vi "GetInfoForVIParser.vi"(5 "Data Types":string[](array[string]), 6 "OutputIdx":i32[](array[numeric]), 7 "InputIdx":i32[](array[numeric]), 8 "Dirs":T1[](array[typedef]), 9 "Param Names":string[](array[string])) -> (0 "OutputIdx Out":i32[](array[numeric]), 1 "InputIdx Out":i32[](array[numeric]), 2 "Dirs Out":T1[](array[typedef]), 3 "ParamNames Out":string[](array[string]), 4 "DataTypesOut":string[](array[string]))   [LabVIEW 2020]
uses:
  <vilib>/AppBuilder/IOStatus.ctl
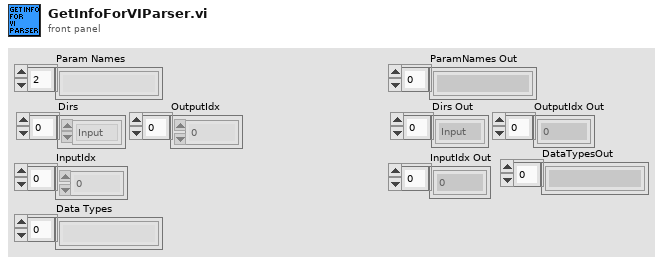
[diagram p1: front panel]
types:
  T1 = typedef "IOStatus.ctl" = enum16{"Input", "Output", "Input/Output", "InputDeleted", "OutputDeleted", "IODeleted", "ErrorClusterIn", "ErrorClusterOut"}
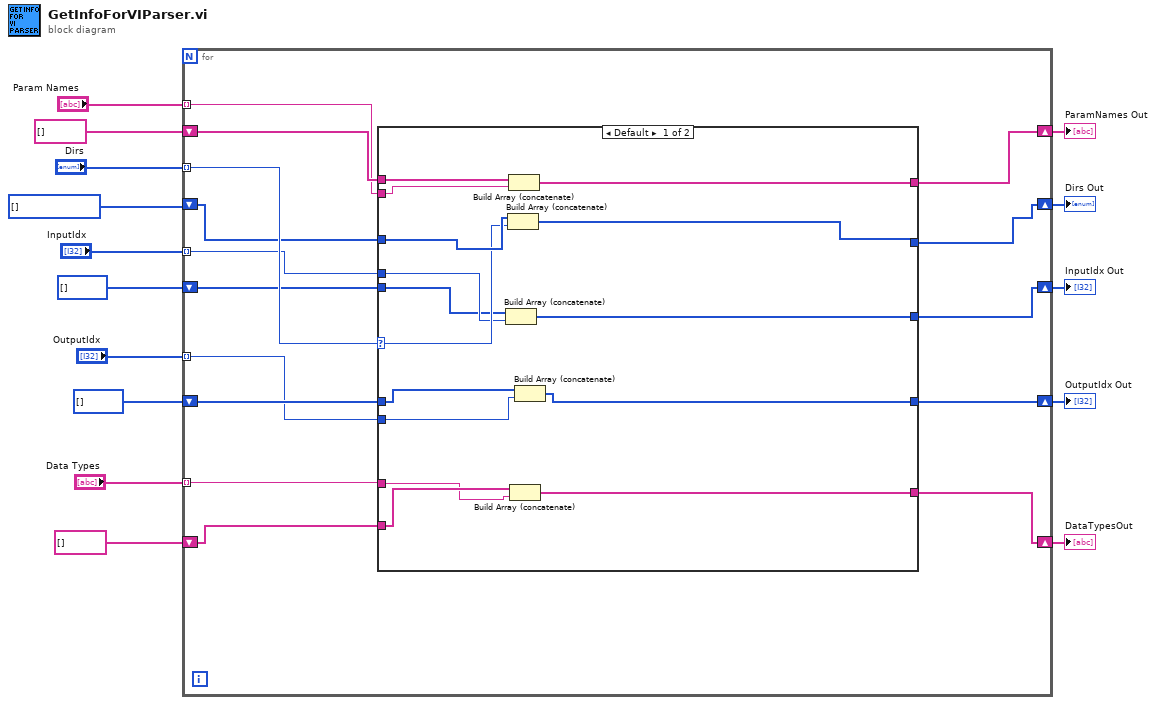
[diagram p0: block diagram]
diagram:
  w6 = T1[] [] items=["Input", "Output", "Input/Output", "InputDeleted", "OutputDeleted", "IODeleted", "ErrorClusterIn", "ErrorClusterOut"] ("Dirs")
  n1 = for {
    tunnel: "Param Names" -> [w28] mode=indexing
    shift-right: [w20] -> w5
    shift-left: string[] [] -> [w29]
    tunnel: "Dirs" -> [w30] mode=indexing
    shift-right: [w19] -> w4
    shift-left: w6 -> [w27]
    tunnel: "InputIdx" -> [w26] mode=indexing
    shift-right: [w18] -> w3
    shift-left: i32[] [] -> [w25]
    shift-right: [w17] -> w2
    shift-left: i32[] [] -> [w24]
    tunnel: "OutputIdx" -> [w23] mode=indexing
    tunnel: "Data Types" -> [w22] mode=indexing
    shift-right: [w16] -> w1
    shift-left: string[] [] -> [w21]
    n2 = case shown="Default" w30 {
      selector: w30 -> [w43 _]
      tunnel: w29 -> [w45 w50]
      tunnel: w28 -> [w31 _]
      tunnel: w27 -> [w44 w49]
      tunnel: w26 -> [w42 _]
      tunnel: w25 -> [w41 w48]
      tunnel: w24 -> [w40 w47]
      tunnel: w23 -> [w39 _]
      tunnel: w22 -> [w37 _]
      tunnel: w21 -> [w38 w46]
      tunnel: [w36 w50] -> w20
      tunnel: [w35 w49] -> w19
      tunnel: [w34 w48] -> w18
      tunnel: [w33 w47] -> w17
      tunnel: [w32 w46] -> w16
      frame Default {
        n3 = Build Array (concatenate)(w41, w42) -> (w34:i32[])
        n4 = Build Array (concatenate)(w44, w43) -> (w35:T1[])
        n5 = Build Array (concatenate)(w45, w31) -> (w36:string[])
        n6 = Build Array (concatenate)(w38, w37) -> (w32:string[])
        n7 = Build Array (concatenate)(w40, w39) -> (w33:i32[])
      }
      frame "InputDeleted".."ErrorClusterIn" {
      }
    }
  }
  "ParamNames Out" <- w5
  "Dirs Out" <- w4
  "InputIdx Out" <- w3
  "OutputIdx Out" <- w2
  "DataTypesOut" <- w1
